vi "from epoch time.vi"() -> ()   [LabVIEW 2020]
panel:
  out "current time":timestamp=timestamp(3029526000 s since 1904-01-01)
  in  "timestamp":u32=654466209
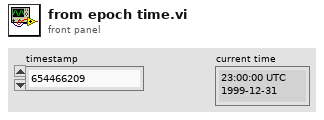
[diagram p1: front panel]
types:
  T1 = typedef "LVDateTimeRec.ctl" = cluster{"fractional second":dbl, "second":i32, "minute":i32, "hour":i32, "day of month":i32, "month":i32, "year":i32, "day of week":i32, "day of year":i32, "DST":i32}
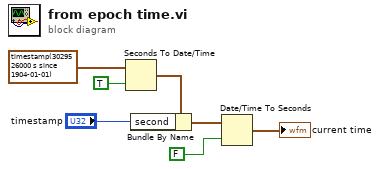
[diagram p0: block diagram]
diagram:
  n1 = Seconds To Date/Time(time stamp (now)=timestamp(3029526000 s since 1904-01-01) ("current time"), to UTC (F)=TRUE) -> (date time rec=w6:T1)
  n2 = Bundle By Name(cluster=w6, "second"="timestamp") -> (w4:T1)
  n3 = Date/Time To Seconds(1:FALSE ("to UTC (F)"), 2:w4) -> (0:→"current time":timestamp)
